vi "Read 1 Hand Position Velocity.vi"(8 "Error In":errorcluster, 11 "Leap Handle":T1) -> (0 "Error Out":errorcluster, 1 "Hand Velocity":cluster{"X":sgl, "Y":sgl, "Z":sgl}, 2 "Hand Position":cluster{"X":sgl, "Y":sgl, "Z":sgl}, 3 "Leap Handle":T1)   [LabVIEW 2011, in "LMH-Leap.lvlib"]
doc: "Read the position and velocity of one hand object in the frame."
uses:
  LMH-Leap.lvlib
  Private/Type Defs/Leap Handle.ctl
  C:/github/makerhub/Leap/LabVIEW/vi.lib/MakerHub/Leap/Private/Libs/LeapCSharp.NET3.5.dll
  Private/Libs/LeapCSharp.NET3.5.dll
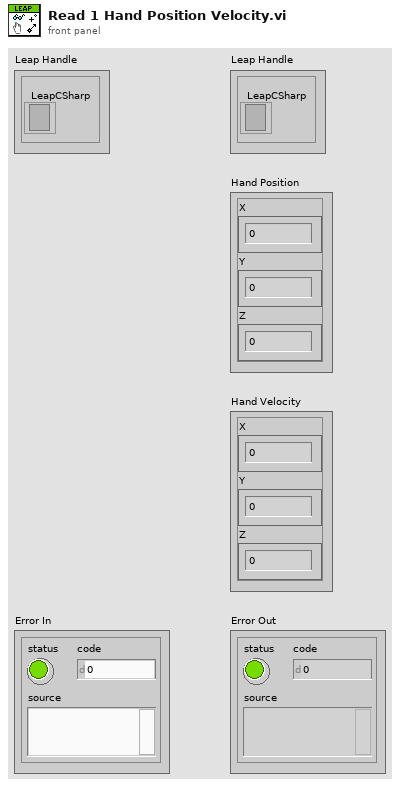
[diagram p1: front panel]
types:
  T1 = typedef "LMH-Leap.lvlib/Leap Handle.ctl" = cluster{"LeapCSharp":refnum<k24>}
  T2 = typedef "LMH-Leap.lvlib/Frame.ctl" = cluster{"ID":i64, "Timestamp":i64, "Current FPS":dbl, "Key Tap Gestures":T3[], "Circle Gestures":T8[], "Screen Tap Gestures":T9[], "Swipe Gestures":T10[], "Hands":T11[]}
  T3 = typedef "LMH-Leap.lvlib/Gesture Key Tap.ctl" = cluster{"Common":T4, "Direction":T7, "Position":T7, "Progress":dbl}
  T4 = typedef "LMH-Leap.lvlib/Gesture Common.ctl" = cluster{"ID":dbl, "Duration (S)":dbl, "Gesture Type":T5, "Gesture State":T6}
  T5 = typedef "LMH-Leap.lvlib/Gesture Type.ctl" = enum16{"Invalid", "Swipe", "Circle", "Screen Tap", "Key Tap"}
  T6 = typedef "LMH-Leap.lvlib/Gesture State.ctl" = enum16{"Invalid", "Start", "Update", "Stop"}
  T7 = typedef "LMH-Leap.lvlib/Vector.ctl" = cluster{"Pitch":sgl, "Yaw":sgl, "Roll":sgl, "Magnitude":sgl, "XYZ":sgl[]}
  T8 = typedef "LMH-Leap.lvlib/Gesture Circle.ctl" = cluster{"Common":T4, "Center":T7, "Normal":T7, "Progress":dbl, "Radius":dbl}
  T9 = typedef "LMH-Leap.lvlib/Gesture Screen Tap.ctl" = cluster{"Common":T4, "Direction":T7, "Position":T7, "Progress":dbl}
  T10 = typedef "LMH-Leap.lvlib/Gesture Swipe.ctl" = cluster{"Common":T4, "Direction":T7, "Position":T7, "Start Position":T7, "Speed":dbl}
  T11 = typedef "LMH-Leap.lvlib/Hand.ctl" = cluster{"Palm Normal":T7, "Palm Position":T7, "Palm Velocity":T7, "Direction":T7, "Palm Position (Stabilized)":T7, "Sphere Center":T7, "Pointables":T12[], "ID":i32, "Time Visible":sgl, "Sphere Radius":sgl}
  T12 = typedef "LMH-Leap.lvlib/Pointable.ctl" = cluster{"Type":T13, "Touch Zone":T14, "ID":i32, "Length":dbl, "Width":dbl, "Time Visible":dbl, "Touch Distance":dbl, "Direction":T7, "Tip Position":T7, "Tip Velocity":T7, "Tip Position (Stabilized)":T7}
  T13 = typedef "LMH-Leap.lvlib/Pointable Type.ctl" = enum16{"Finger", "Tool"}
  T14 = typedef "LMH-Leap.lvlib/Pointable Zone.ctl" = enum16{"None", "Hovering", "Touching"}
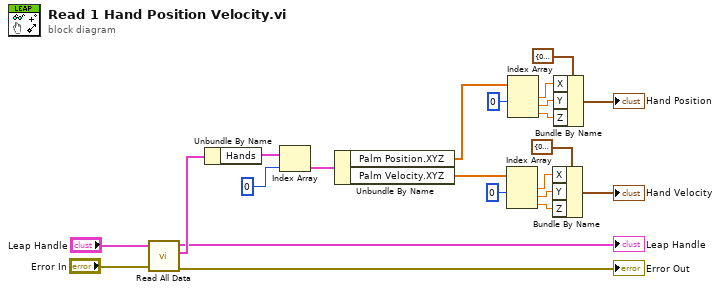
[diagram p0: block diagram]
diagram:
  n1 = call "Read All Data.vi"("Error In"="Error In", "Leap Handle"="Leap Handle") -> ("Error Out"=→"Error Out":errorcluster, "Frame"=w20:T2, "Leap Handle"=→"Leap Handle":T1)  [unwired: 6 in, 1 out]
  n2 = Unbundle By Name(w20) -> ("Hands"=w4:T11[])
  n3 = Index Array(array=w4, index=0) -> (element=w3:T11)
  n4 = Unbundle By Name(w3) -> ("Palm Position.XYZ"=w16:sgl[], "Palm Velocity.XYZ"=w6:sgl[])
  n5 = Index Array(array=w6, index #1=0 ("index")) -> (element #1=w9:sgl, element #2=w10:sgl, element #3=w11:sgl)  [unwired: 2 in]
  n6 = Index Array(array=w16, index #1=0 ("index")) -> (element #1=w14:sgl, element #2=w13:sgl, element #3=w12:sgl)  [unwired: 2 in]
  n7 = Bundle By Name(cluster=cluster{"X":sgl, "Y":sgl, "Z":sgl} {"X"=0.0, "Y"=0.0, "Z"=0.0}, "X"=w9, "Y"=w10, "Z"=w11) -> (→"Hand Velocity":cluster{"X":sgl, "Y":sgl, "Z":sgl})
  n8 = Bundle By Name(cluster=cluster{"X":sgl, "Y":sgl, "Z":sgl} {"X"=0.0, "Y"=0.0, "Z"=0.0}, "X"=w14, "Y"=w13, "Z"=w12) -> (→"Hand Position":cluster{"X":sgl, "Y":sgl, "Z":sgl})
